vi "RC_MoveTable.vi"(7 "Index":dbl, 8 "ID":dbl, 10 "CMD":dbl) -> (1 "Value":i32, 3 "RC ID":i32)   [LabVIEW 2018]
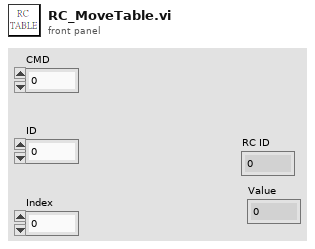
[diagram p1: front panel]
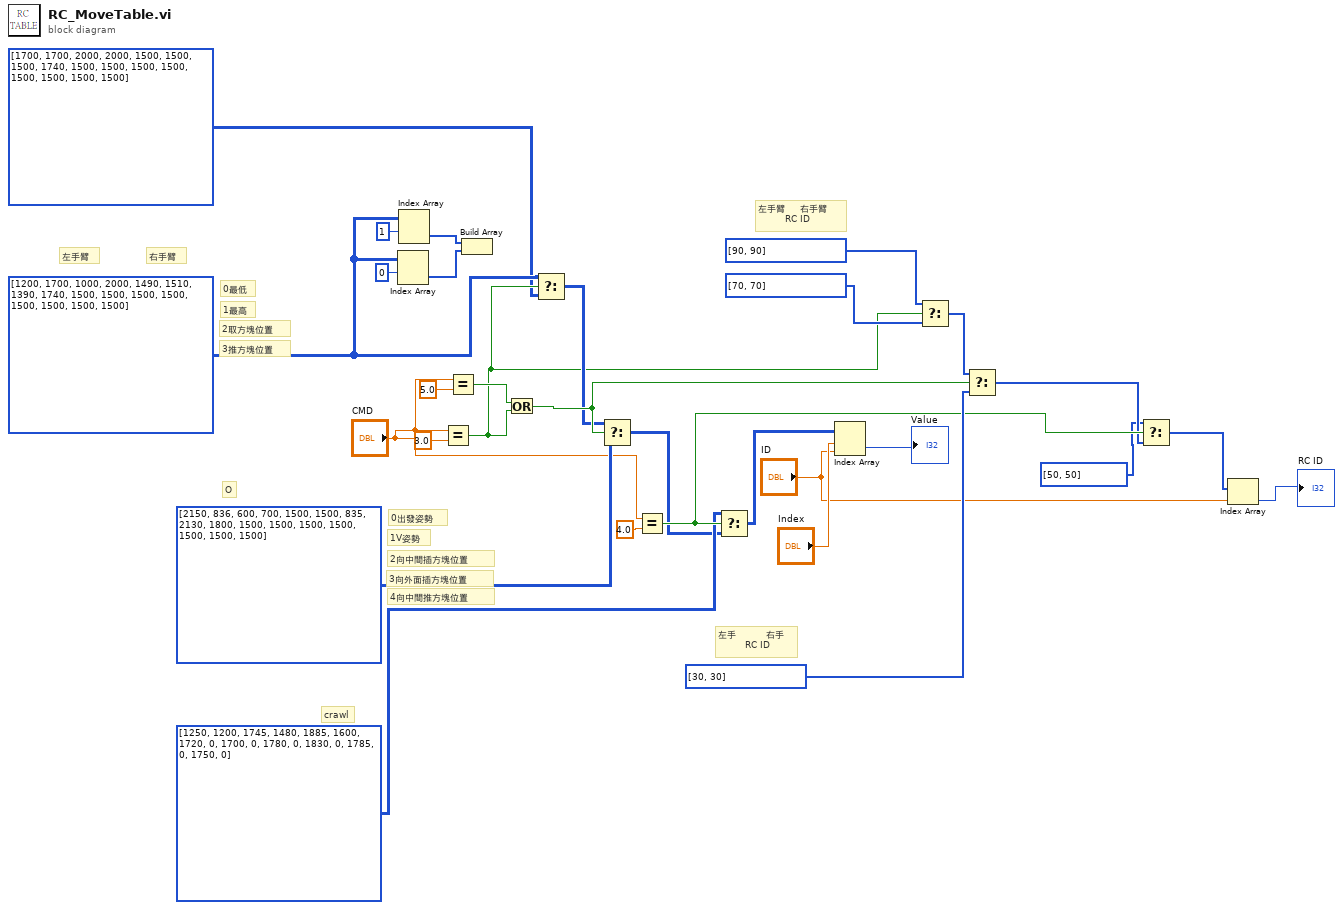
[diagram p0: block diagram]
diagram:
  w2 = i32[][] [[1200, 1700], [1000, 2000], [1490, 1510], [1390, 1740], [1500, 1500], [1500, 1500], [1500, 1500], [1500, 1500]]
  # "O"
  # "crawl"
  # "左手          右手\n         RC ID"
  # "左手臂     右手臂\n         RC ID"
  # "4向中間推方塊位置"
  # "3向外面插方塊位置"
  # "2向中間插方塊位置"
  # "1V姿勢"
  # "0出發姿勢"
  # "3推方塊位置"
  # "2取方塊位置"
  # "1最高"
  # "0最低"
  # "右手臂"
  # "左手臂"
  n1 = Index Array(array=w2, index (row)=0) -> (element=w5:i32[])  [unwired: 1 in]
  n2 = Index Array(array=w2, index (row)=1) -> (element=w6:i32[])  [unwired: 1 in]
  n3 = Equal?(x="CMD", y=3.0) -> (x = y?=w3:bool)
  n4 = Equal?(x="CMD", y=5.0) -> (x = y?=w13:bool)
  n5 = Build Array(w6, w5) -> ()  [unwired: 1 out]
  n6 = Or(x=w13, y=w3) -> (x .or. y?=w14:bool)
  n7 = Select(t=w2, s=w3, f=i32[][] [[1700, 1700], [2000, 2000], [1500, 1500], [1500, 1740], [1500, 1500], [1500, 1500], [1500, 1500], [1500, 1500]]) -> (s? t:f=w4:i32[][])
  n8 = Select(t=w4, s=w14, f=i32[][] [[2150, 836], [600, 700], [1500, 1500], [835, 2130], [1800, 1500], [1500, 1500], [1500, 1500], [1500, 1500]]) -> (s? t:f=w19:i32[][])
  n9 = Equal?(x="CMD", y=4.0) -> (x = y?=w22:bool)
  n10 = Select(t=i32[][] [[1250, 1200], [1745, 1480], [1885, 1600], [1720, 0], [1700, 0], [1780, 0], [1830, 0], [1785, 0], [1750, 0]], s=w22, f=w19) -> (s? t:f=w23:i32[][])
  n11 = Index Array(array=w23, index (row)="Index", index (col)="ID") -> (element=→"Value":i32)
  n12 = Select(t=i32[] [90, 90], s=w3, f=i32[] [70, 70]) -> (s? t:f=w7:i32[])
  n13 = Select(t=w7, s=w14, f=i32[] [30, 30]) -> (s? t:f=w18:i32[])
  n14 = Select(t=i32[] [50, 50] ("f"), s=w22, f=w18) -> (s? t:f=w21:i32[])
  n15 = Index Array(array=w21, index="ID") -> (element=→"RC ID":i32)
